vi "Math Rolling Buffer.vi"(0 "New Data In":sgl[][](array[numeric]), 1 "# Pts Read":u32, 3 "Number of Channels":i32=1, 4 "Sample Rate":dbl=2000.0, 5 "error in (no error)":errorcluster, 6 "Math Rolling Buffer Ref":refnum<vi>, 7 "Config.Test Limits":T1[](array[typedef]), 9 "Coefficients":cluster{"Coefficients":dbl[]}[](array[cluster]), 10 "Mode (Read)":T2=enum."Read") -> (14 "Buffer Out":sgl[][](array[numeric]), 15 "Data Indexes":i32[](array[numeric]), 16 "RMS":sgl[][](array[numeric]), 17 "PK-PK":sgl[][](array[numeric]), 18 "Frequency Data":sgl[][](array[numeric]), 19 "error out":errorcluster)   [LabVIEW 2019]
uses:
  Type Defs and Controls/Functional Global Control.ctl
  Type Defs and Controls/Test Limits.ctl
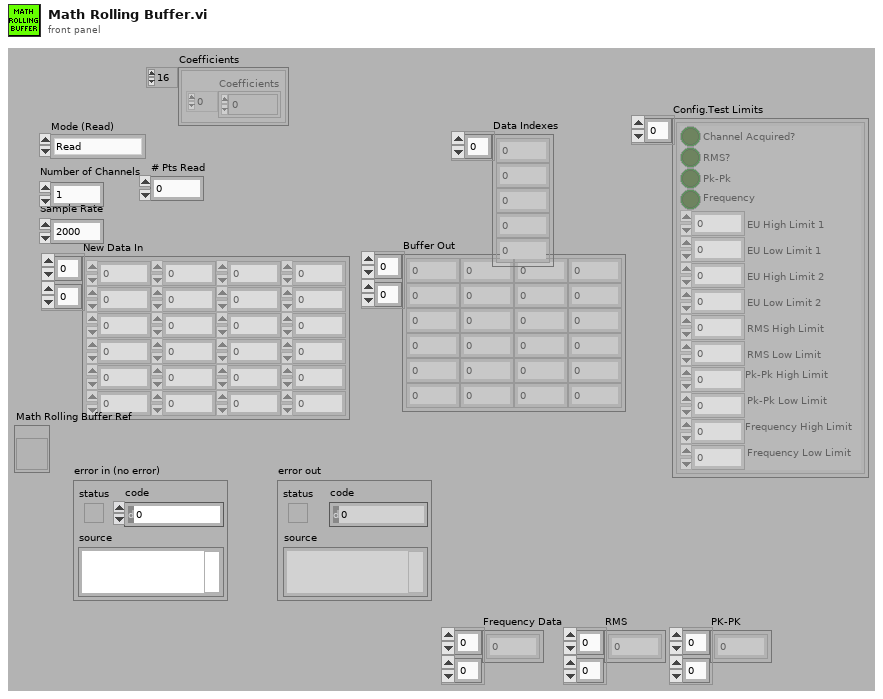
[diagram p1: front panel]
types:
  T1 = typedef "Test Limits.ctl" = cluster{"Channel Acquired?":bool, "RMS?":bool, "Pk-Pk":bool, "Frequency":bool, "EU High Limit 1":dbl, "EU Low Limit 1":dbl, "EU High Limit 2":dbl, "EU Low Limit 2":dbl, "RMS High Limit":dbl, "RMS Low Limit":dbl, "Pk-Pk High Limit ":dbl, "Pk-Pk Low Limit":dbl, "Frequency High Limit":dbl, "Frequency Low Limit":dbl}
  T2 = typedef "Functional Global Control.ctl" = enum16{"Nothing", "Init", "Read", "Write"}
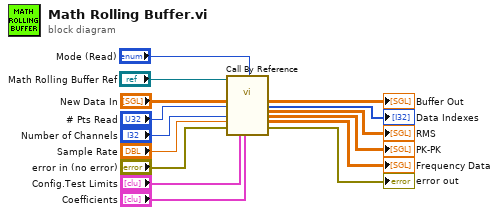
[diagram p0: block diagram]
diagram:
  n1 = call-by-ref "?"(reference="Math Rolling Buffer Ref", "New Data In"="New Data In", "# Pts Read"="# Pts Read", "Number of Channels"="Number of Channels", "Sample Rate"="Sample Rate", "error in (no error)"="error in (no error)", "Config.Test Limits"="Config.Test Limits", "Coefficients"="Coefficients", "Mode (Read)"="Mode (Read)") -> ("Buffer Out"=→"Buffer Out":sgl[][], "Data Indexes"=→"Data Indexes":i32[], "RMS"=→"RMS":sgl[][], "PK-PK"=→"PK-PK":sgl[][], "Frequency Data"=→"Frequency Data":sgl[][], "error out"=→"error out":errorcluster)  [unwired: 7 in, 2 out]
